vi "Master network read write.vi"(7 "Modbus master in":refnum<class "Modbus Master.lvclass">, 8 "error in":errorcluster, 9 "transmission data unit in":refnum<class "Transmission Data Unit.lvclass">, 10 "network master in":refnum<class "Network Master.lvclass">, 11 "Modbus data unit in":refnum<class "Modbus Data Unit.lvclass">) -> (0 "error out":errorcluster, 1 "transmission data unit out":refnum<class "Transmission Data Unit.lvclass">, 2 "PDU Valid?":bool, 3 "Modbus data unit out":refnum<class "Modbus Data Unit.lvclass">, 5 "Modbus master out":refnum<class "Modbus Master.lvclass">)   [LabVIEW 2013, in "Modbus Library - Advance.lvlib" / "Modbus Master.lvclass"]
doc: "This VI allows a mutex for the master API without restricting any other functions. This mutex is currently unimplemented."
uses:
  Modbus Master.lvclass
  Network Protocol/Network Master/Network Master.lvclass
  Transmission Data Unit/Transmission Data Unit.lvclass
  Modbus Data Unit/Modbus Data Unit.lvclass
  Modbus Master.lvclass/Modbus Master.ctl
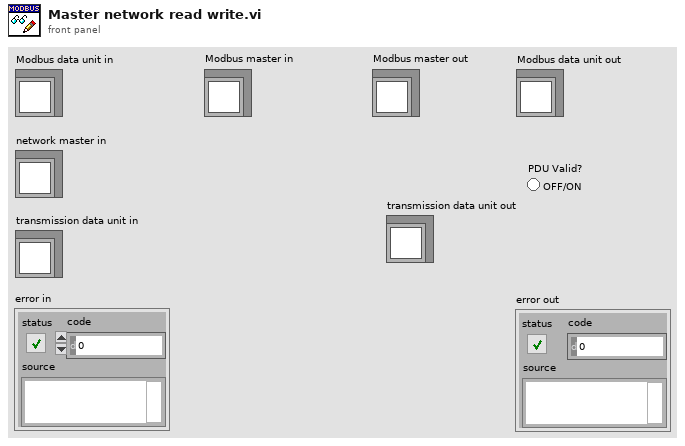
[diagram p1: front panel]
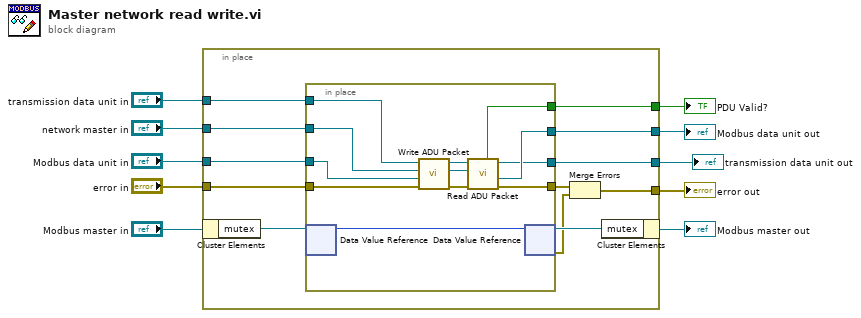
[diagram p0: block diagram]
diagram:
  n1 = in-place {
    in-place-border: "error in" -> [w21]
    in-place-border: "Modbus data unit in" -> [w20]
    in-place-border: "transmission data unit in" -> [w18]
    in-place-border: "network master in" -> [w17]
    in-place-border: [w14] -> w4
    in-place-border: [w13] -> w3
    in-place-border: [w12] -> w2
    in-place-border: [w11] -> w1
    n2 = in-place-cluster #1("Modbus master in") -> ("mutex"=w22:refnum<data-value>)
    n3 = in-place {
      in-place-border: w21 -> [w30]
      in-place-border: w20 -> [w29]
      in-place-border: w18 -> [w28]
      in-place-border: w17 -> [w26]
      in-place-border: [w27] -> w16
      in-place-border: [w25] -> w14
      in-place-border: [w24] -> w12
      in-place-border: [w23] -> w11
      n4 = in-place-dvr #2(w22) -> (w31:u8)  [unwired: 1 out]
      n5 = call-dynamic "Write ADU Packet.vi"("error in"=w30, "modbus data unit"=w29, "protocol layer"=w26, "transmission data unit in"=w28) -> ("error out"=w33:errorcluster, "protocol layer out"=w34:refnum<class "Network Protocol.lvclass">, "transmission data unit out"=w32:refnum<class "Transmission Data Unit.lvclass">)  [unwired: 5 in]
      n6 = call-dynamic "Read ADU Packet.vi"("error in"=w33, "protocol layer"=w34, "transmission data unit in"=w32) -> ("error out"=w27:errorcluster, "modbus data unit"=w25:refnum<class "Modbus Data Unit.lvclass">, "transmission data unit out"=w23:refnum<class "Transmission Data Unit.lvclass">, "PDU Valid?"=w24:bool)  [unwired: 4 in, 1 out]
      n7 = in-place-dvr #2(w31) -> (w19:refnum<data-value>, w15:errorcluster)
    }
    n8 = Merge Errors(w16, w15) -> (w13:errorcluster)
    n9 = in-place-cluster #1("mutex"=w19) -> (→"Modbus master out":refnum<class "Modbus Master.lvclass">)
  }
  "Modbus data unit out" <- w4
  "error out" <- w3
  "PDU Valid?" <- w2
  "transmission data unit out" <- w1
